vi "Target VI Path.vi"(1 "Instrument Name":string) -> (0 "Path to VI":path)   [LabVIEW 2015]
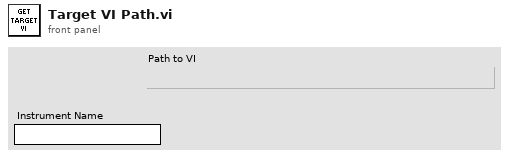
[diagram p1: front panel]
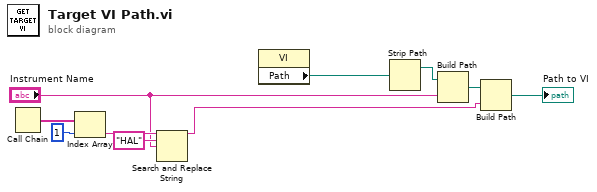
[diagram p0: block diagram]
diagram:
  n1 = Call Chain() -> (call chain=w10:string[])
  n2 = Index Array(array=w10, index=1) -> (element=w7:string)
  n3 = Search and Replace String(input string=w7, search string="HAL", replace string="Instrument Name") -> (result string=w4:string)  [unwired: 5 in, 3 out]
  n4 = property class="VI"() -> ("Path"=w1:path)  [unwired: 2 in, 2 out]
  n5 = Strip Path(path=w1) -> (stripped path=w3:path)  [unwired: 1 out]
  n6 = Build Path(base path=w3, name or relative path="Instrument Name") -> (appended path=w2:path)
  n7 = Build Path(base path=w2, name or relative path=w4) -> (appended path=→"Path to VI":path)
